vi "Update Connected Clients.vi"(8 "error in (no error)":errorcluster, 10 "2D Array of String":string[][](array[string]), 11 "Function in":refnum<class "Function.lvclass">) -> (0 "error out":errorcluster, 3 "Function out":refnum<class "Function.lvclass">)   [LabVIEW 2016, in "Function Actor.lvlib" / "Function.lvclass"]
uses:
  <userlib>/Common Components/Function Actor/Function.lvclass
  <userlib>/Common Components/Function Actor/Function.lvclass/Function.ctl
  <userlib>/Common Components/Common/Connected Client Cluster.ctl
  <userlib>/Common Components/Common/Common.lvlib
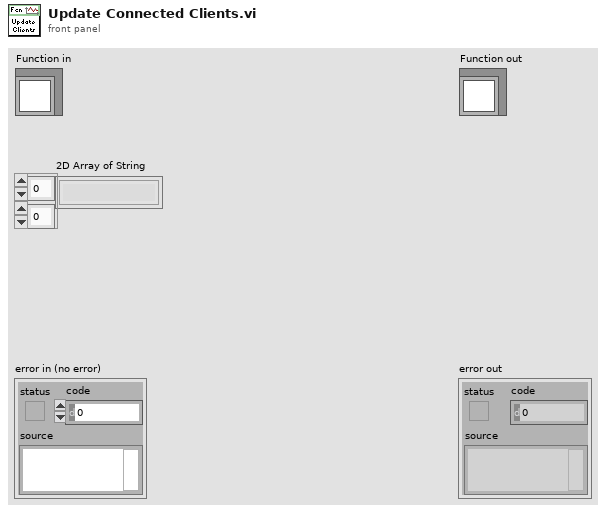
[diagram p1: front panel]
types:
  T1 = typedef "Common.lvlib/Connected Client Cluster.ctl" = cluster{"IP Address":string, "Username":string, "Access Level":string}
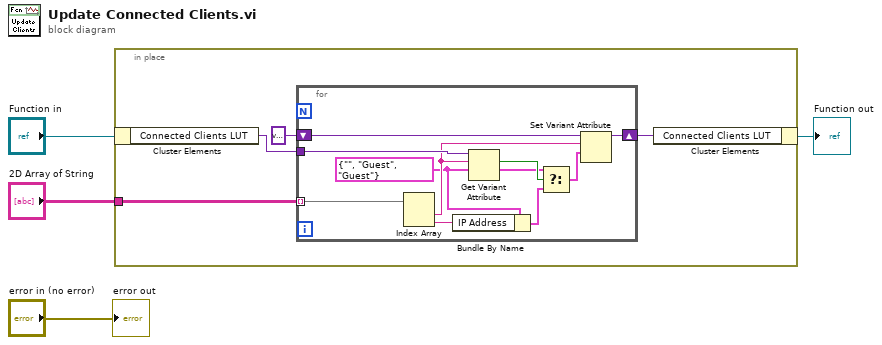
[diagram p0: block diagram]
diagram:
  n1 = in-place {
    in-place-border: "2D Array of String" -> [w8]
    n2 = in-place-cluster #1("Function in") -> ("Connected Clients LUT"=w7:variant)
    n3 = for {
      tunnel: w8 -> [w19] mode=indexing
      tunnel: w7 -> [w18]
      shift-right: [w17] -> w6
      shift-left: variant -> [w13]
      w15 = T1 {"IP Address"="", "Username"="Guest", "Access Level"="Guest"} ("Connected Client Cluster")
      n4 = Index Array(array=w19) -> (element #1=w16:string, element #2=w14:string)  [unwired: 2 in]
      n5 = Bundle By Name(cluster=w15, "IP Address"=w14) -> (w10:T1)
      n6 = Get Variant Attribute(Variant=w18, name=w16, default value (empty Variant)=w15) -> (found=w12:bool, value=w11:T1)  [unwired: 1 in, 2 out]
      n7 = Select(t=w11, s=w12, f=w10) -> (s? t:f=w9:T1)
      n8 = Set Variant Attribute(Variant=w13, name=w16, value=w9) -> (Variant out=w17:variant)  [unwired: 1 in, 2 out]
    }
    n9 = in-place-cluster #1("Connected Clients LUT"=w6) -> (→"Function out":refnum<class "Function.lvclass">)
  }
  "error out" <- "error in (no error)"
